vi "TecanCarvroPump_Basic.vi"(0 "TecanPump COM":refnum<visa-resource-name>="COM6", 1 "Volume (μL)":u16=30, 2 "急停":bool, 5 "TecanPump address":u8=1 max=16 step=1, 7 "Valve":u8(knob)=2 max=6 step=1 scale=1.0..3.0, 9 "Mode":T1(ring)=enum."Relative Dispense", 11 "Syringe size (μL)":u16=1000 min=1 max=5000 step=1, 12 "Speed (μL/s)":u16=20 min=1 max=5000 step=1) -> (4 "Input string":string)   [LabVIEW 2023]
panel:
  out "错误输出":errorcluster
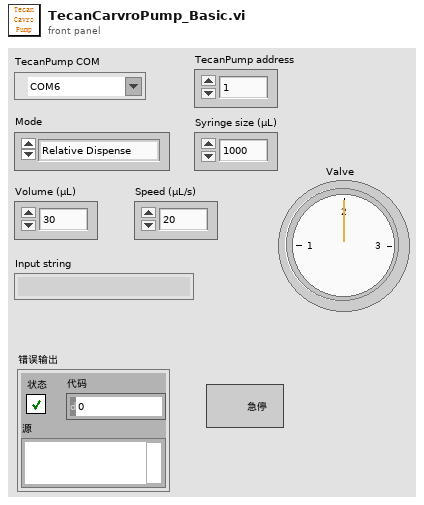
[diagram p1: front panel]
types:
  T1 = enum16{"Initialize", "Absolute Position", "Relative Pickup", "Relative Dispense", "Swich valve", "Bypass"}
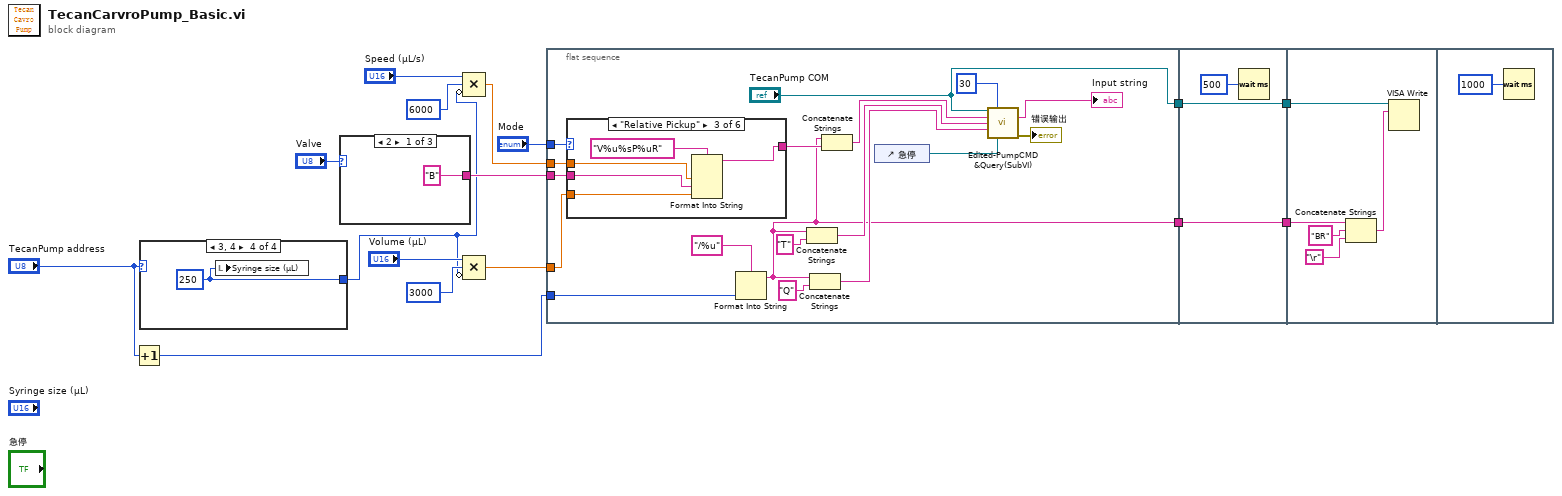
[diagram p0: block diagram]
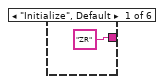
[diagram p2: hidden frame]
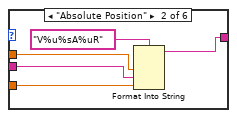
[diagram p3: hidden frame]
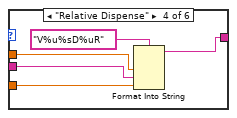
[diagram p4: hidden frame]
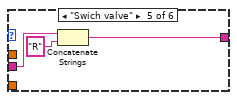
[diagram p5: hidden frame]
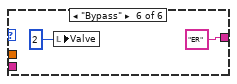
[diagram p6: hidden frame]
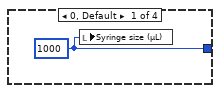
[diagram p7: hidden frame]
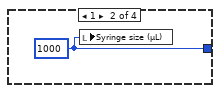
[diagram p8: hidden frame]
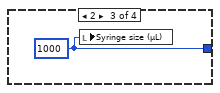
[diagram p9: hidden frame]
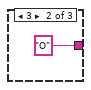
[diagram p10: hidden frame]
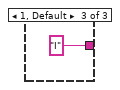
[diagram p11: hidden frame]
diagram:
  n1 = Increment(x="TecanPump address") -> (x+1=w16:u8)
  n2 = case shown="3, 4" "TecanPump address" {
    tunnel: [w17 w18 w19 w20] -> w6
    frame 0, Default {
      w17 = u16 1000 ("Syringe size (μL)")
      n3 = local write "Syringe size (μL)"(w17) -> ()
    }
    frame 1 {
      w18 = u16 1000 ("Syringe size (μL)")
      n4 = local write "Syringe size (μL)"(w18) -> ()
    }
    frame 2 {
      w19 = u16 1000 ("Syringe size (μL)")
      n5 = local write "Syringe size (μL)"(w19) -> ()
    }
    frame 3, 4 {
      w20 = u16 250 ("Syringe size (μL)")
      n6 = local write "Syringe size (μL)"(w20) -> ()
    }
  }
  n7 = case shown="2" "Valve" {
    tunnel: ["B" ("format string") "O" ("format string") "I" ("format string")] -> w8
    frame 2 {
    }
    frame 3 {
    }
    frame 1, Default {
    }
  }
  n8 = Compound Arithmetic op=MULTIPLY("Speed (μL/s)", u16 6000 ("value"), invert w6) -> (w9:dbl)
  n9 = Compound Arithmetic op=MULTIPLY("Volume (μL)", u16 3000 ("value"), invert w6) -> (w14:dbl)
  n10 = flat-sequence {
    tunnel: w16 -> [w32]
    tunnel: "Mode" -> [w31]
    tunnel: w14 -> [w30]
    tunnel: w9 -> [w29]
    tunnel: w8 -> [w27]
    tunnel: [w25] -> w4
    tunnel: ["TecanPump COM"] -> w2
    tunnel: w4 -> [w65]
    tunnel: [w65] -> w3
    tunnel: w2 -> [w64]
    tunnel: [w64] -> w1
    tunnel: w3 -> [w69]
    tunnel: w1 -> [w66]
    frame #0 {
      n11 = case shown="\"Relative Pickup\"" w31 {
        tunnel: w30 -> [_ w43 w50 w55 _ _]
        tunnel: w29 -> [_ w46 w51 w56 _ _]
        tunnel: ["ZR" w45 w48 w53 w58 "ER" ("string")] -> w28
        tunnel: w27 -> [_ w44 w49 w54 w60 _]
        frame "Initialize", Default {
        }
        frame "Absolute Position" {
          n12 = Format Into String(format string="V%u%sA%uR", w46, w44, w43) -> (resulting string=w45:string)  [unwired: 2 in, 1 out]
        }
        frame "Relative Pickup" {
          n13 = Format Into String(format string="V%u%sP%uR", w51, w49, w50) -> (resulting string=w48:string)  [unwired: 2 in, 1 out]
        }
        frame "Relative Dispense" {
          n14 = Format Into String(format string="V%u%sD%uR", w56, w54, w55) -> (resulting string=w53:string)  [unwired: 2 in, 1 out]
        }
        frame "Swich valve" {
          n15 = Concatenate Strings(w60, "R" ("string")) -> (w58:string)
        }
        frame "Bypass" {
          n16 = local write "Valve"(u8 2 ("Valve")) -> ()
        }
      }
      n17 = Format Into String(format string="/%u" ("字符串"), w32) -> (resulting string=w25:string)  [unwired: 2 in, 1 out]
      n18 = Concatenate Strings(w25, "T" ("字符串")) -> (w36:string)
      n19 = Concatenate Strings(w25, "Q" ("字符串")) -> (w35:string)
      n20 = Concatenate Strings(w25, w28) -> (w37:string)
      n21 = control-ref of="急停"() -> (w26:refnum<vi>)
      n22 = call "Edited-PumpCMD&Query(SubVI).vi"("VISA资源名称"="TecanPump COM", "允许执行时间"=u32 30, "命令"=w37, "急停"=w36, "查询"=w35, "emergence"=w26) -> ("Input string"=→"Input string":string, "错误输出"=→"错误输出":errorcluster)  [unwired: 7 in, 1 out]
    }
    frame #1 {
      n23 = Wait (ms)(milliseconds to wait=u32 500) -> ()  [unwired: 1 out]
    }
    frame #2 {
      n24 = Concatenate Strings(w69, "BR" ("format string"), "\r") -> (w67:string)
      n25 = VISA Write(VISA resource name=w66, write buffer=w67) -> ()  [unwired: 1 in, 3 out]
    }
    frame #3 {
      n26 = Wait (ms)(milliseconds to wait=u32 1000) -> ()  [unwired: 1 out]
    }
  }
